vi "3_2_Objects_Detection(Deploy)(Cam).vi"() -> ()   [LabVIEW 2020]
doc: "This example demonstrates usage of Deep Learning Toolkit for object detection based on pretrained network called YOLO https://pjreddie.com/darknet/yolo/\nToolkit's API is utilized to automatically create network architecture based on network topology configuration file and load and initialize network's weights from weight file.\nRequirements: \n1. Deep Learning Toolkit for LabVIEW.\n2. NI Vision Development Module .\n3. Web camera."
uses:
  <vilib>/Ngene/Deep Learning Toolkit/Toolkit/NN_Network/Controls/NN_Device.ctl
  <vilib>/Ngene/Deep Learning Toolkit/Toolkit/NN_Network/Controls/NN_Save_Before_Destroy_Options.ctl
  <vilib>/vision/driver/IMAQdx.llb/IMAQdx Camera Control Mode.ctl
  <vilib>/Ngene/Deep Learning Toolkit/Toolkit/Utils/Vision/Coords_Rect2PolyLine.vi
  <vilib>/Ngene/Deep Learning Toolkit/Toolkit/NN_Network/API/NN_Set_Input/3D/NN_Set_Input(3D_SGL_idx).vi
  <vilib>/Ngene/Deep Learning Toolkit/Toolkit/Deep_Learning_Toolkit_by_Ngene.lvlib
  <vilib>/vision/NI_Vision_Development_Module.lvlib
  <vilib>/vision/driver/NI_Vision_Acquisition_Software.lvlib
  <resource>/objmgr/imaqdx.rc
  <vilib>/ptbypt/NI_PtbyPt.lvlib
panel:
  in  "NN_Device":T1
  out "Speed (FPS)":dbl format="%#_3p"
  out "Loop time(s)":dbl format="%#_3p"
  out "Display":T2(plugin-control)
  in  "Confidence_Thresh":sgl=0.19999999
  in  "IOU_Thresh(NMS)":sgl=0.3
  in  "Stop":bool
  in  "Camera Resolution":i32(listbox)=14
  in  "Camera":refnum<k21>="cam0" caption="IMAQdx Session"
  in  "Model Weights":path=path "D:/Ngene/GitHub/deepltk_examples/3_Image_Processing/33_Object_Detection/Trained Model/512x910_mAP_0.998/Obj_Det_Example_weights_25_06_09__13_45_53.bin"
  in  "Model Topology (CFG)":path=path "D:/Ngene/GitHub/deepltk_examples/3_Image_Processing/33_Object_Detection/Trained Model/512x910_mAP_0.998/Obj_Det_Example_net_cfg_25_06_09__13_45_53.cfg"
  # "Instructions:\n1.Provide the \"Model Topology (CFG)\" and \"Model Weights\" generated after training in \"Objects_Detection(Train).vi\". A pretrained model is also available in the project.\n2. Select the camera from \"Camera\" control.\n3. Run the VI .\n4. Observe the detections drawn on the \"Display\". The info on the top left of each bounding box represents detected object class and the confidence level.\n5. (Optional) Change \"NN_Device\" value to \"GPU\" to compare execution speeds on GPU and CPU.\n\nMore Examples:  https://github.com/ngenehub/deepltk_examples"
  # "Overview:  This example demonstrates the process of deploying an object detection model, capturing samples from a camera, and performing inference.\nRequirements: \n1. Deep Learning Toolkit for LabVIEW.\n2. NI Vision Development Module .\n3. Web camera."
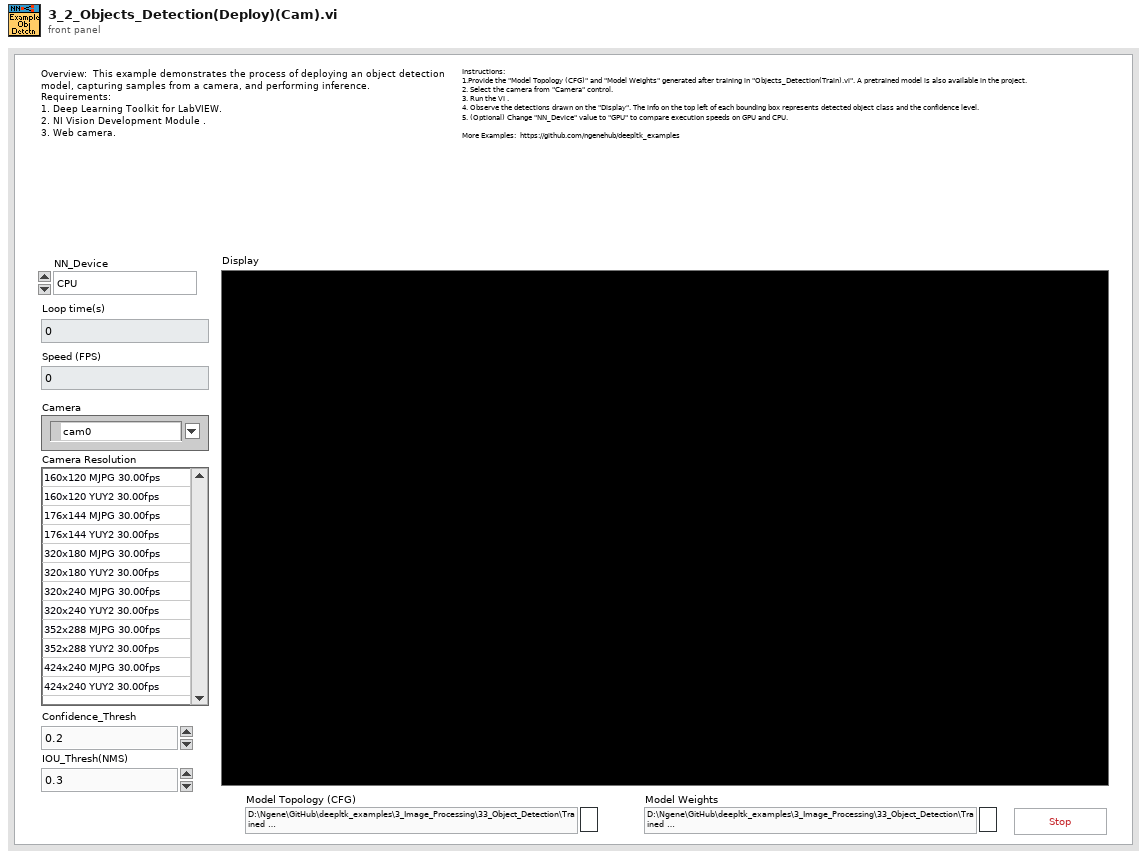
[diagram p1: front panel]
types:
  T1 = typedef "Deep_Learning_Toolkit_by_Ngene.lvlib/NN_Device.ctl" = enum16{"CPU", "GPU"}
  T2 = typedef "IMAQ Image.ctl" = refnum<image>
  T3 = typedef "Deep_Learning_Toolkit_by_Ngene.lvlib/NN_Save_Before_Destroy_Options.ctl" = cluster{"CFG?":bool, "Weights?":bool, "Render?":bool}
  T4 = typedef "NI_Vision_Acquisition_Software.lvlib/IMAQdx Camera Control Mode.ctl" = enum32{"Controller", "Listener"}
  T5 = typedef "Image Type" = u32
  T6 = typedef "IMAQdx.ctl" = refnum<k21>
  T7 = typedef "Deep_Learning_Toolkit_by_Ngene.lvlib/NN_Config_Params.ctl" = cluster{"Name":string, "mBatch":i32, "NN_Train_Params":T8, "LR_Decay_Policy":T11, "Labels":string[], "Loss":T13, "Max_WS_Size(B)":i64, "DryRun?":bool}
  T8 = typedef "Deep_Learning_Toolkit_by_Ngene.lvlib/NN_Train_Params.ctl" = cluster{"Optimizer":T9, "Beta_1":sgl, "Beta_2":sgl, "Weight Decay(L1)":sgl, "Weight Decay(L2)":sgl, "Data_Sampling":T10}
  T9 = typedef "Deep_Learning_Toolkit_by_Ngene.lvlib/NN_Train_Optimizer.ctl" = enum16{"SGD", "Adam", "Adagrad", "Adadelta", "RMSProp", "Nesterov"}
  T10 = typedef "Deep_Learning_Toolkit_by_Ngene.lvlib/NN_Train_Data_Sampling.ctl" = enum16{"Random", "Sequential"}
  T11 = typedef "Deep_Learning_Toolkit_by_Ngene.lvlib/NN_LR_Policy_Cfg.ctl" = cluster{"Policy_Type":T12, "LR0":dbl, "k":sgl, "WarmUp_Policy":enum16{"Step", "Ramp"}, "WarmUp_Iter":i32, "WarmUp_Ratio":sgl}
  T12 = typedef "Deep_Learning_Toolkit_by_Ngene.lvlib/NN_LR_Policy_Type.ctl" = enum16{"Manual", "Step", "Exp", "1/t"}
  T13 = typedef "Deep_Learning_Toolkit_by_Ngene.lvlib/NN_Loss_Config_Params.ctl" = cluster{"Loss_Type":T14, "Loss_Conf_Params":variant}
  T14 = typedef "Deep_Learning_Toolkit_by_Ngene.lvlib/NN_Loss_Type.ctl" = enum16{"None", "MSE", "CrossEntropy", "YOLO_v2", "YOLO_v4"}
  T15 = typedef "Deep_Learning_Toolkit_by_Ngene.lvlib/NN_Layer_Config_Params.ctl" = cluster{"Layer_Type":T16, "Layer_Conf_Params":variant, "Input Layers":string[]}
  T16 = typedef "Deep_Learning_Toolkit_by_Ngene.lvlib/NN_Layer_Type.ctl" = enum16{"Input1D", "Input3D", "Conv1D", "Conv2D", "Conv2D_Adv", "MaxPool", "AvgPool", "UpSample", "DropOut3D", "ShortCut", "Concat", "SoftMax3D", "FC", "DropOut", "Softmax", "Flatten", "YOLO_v2", "YOLO_v4", "Activation", "BatchNormalization", "LayerNormalization", "Scale", "Unsupported"}
  T17 = typedef "Deep_Learning_Toolkit_by_Ngene.lvlib/NN.ctl" = cluster{"Name":string, "No of Layers":i32, "mBatch":i32, "Layers":T18[], "Dimty":T19, "Dims_In":T20, "Dims_Out":T20, "Working_Dir":path, "Train?":bool, "Train_Params":T8, "LR_Update_Policy":T11, "Session Data":T21, "Ground_truth":T22, "NNg_hdls":T23, "NN_Device":T1, "GPU Id":i32, "Labels":string[], "Loss_Type":T14, "Loss_Cfg_Prms":variant, "NNG_WS":T24, "DryRun?":bool}
  T18 = typedef "Deep_Learning_Toolkit_by_Ngene.lvlib/NN_Layer_ref.ctl" = refnum<file>
  T19 = typedef "Deep_Learning_Toolkit_by_Ngene.lvlib/NN_In_Out_Dim-ty.ctl" = enum8{"In1D_Out1D", "In3D_Out1D", "In3D_Out3D", "In3D_OutBBox"}
  T20 = typedef "Deep_Learning_Toolkit_by_Ngene.lvlib/NN_Dims(C,H,W).ctl" = cluster{"C":i32, "H":i32, "W":i32}
  T21 = typedef "Deep_Learning_Toolkit_by_Ngene.lvlib/NN_Train_Session_Data.ctl" = cluster{"Epochs":sgl, "Tot_Iter":i32, "LR":sgl, "LR_iter":i32}
  T22 = typedef "Deep_Learning_Toolkit_by_Ngene.lvlib/NN_Ground_truth.ctl" = cluster{"Y":variant}
  T23 = typedef "Deep_Learning_Toolkit_by_Ngene.lvlib/nng_cuda_handles.ctl" = cluster{"cudnn":u64, "cublas":u64, "stream":u64, "curand":u64}
  T24 = typedef "Deep_Learning_Toolkit_by_Ngene.lvlib/NNG_WS.ctl" = cluster{"NNG_WS_Mem":T25, "Max_WS_Size":i64}
  T25 = typedef "Deep_Learning_Toolkit_by_Ngene.lvlib/NNg_WS_Mem_DVR.ctl" = refnum<data-value>
  T26 = typedef "Deep_Learning_Toolkit_by_Ngene.lvlib/NN_Layer.ctl" = cluster{"Name":string, "Layer_Data":T27, "Layer_Type":T16, "Dims_In":T20, "Layers_In":T18[], "Dims_Out":T20, "Layers_Out":T18[], "Metrics":T28, "GPU_Data":T29, "mBatch":i32, "NN_Device":T1, "NNg_hdls":T23, "Train?":bool, "Dimty":T30, "RecptField":T31, "Idx":i32}
  T27 = typedef "Deep_Learning_Toolkit_by_Ngene.lvlib/NN_Layer_Data_Refnum.ctl" = refnum<file>
  T28 = typedef "Deep_Learning_Toolkit_by_Ngene.lvlib/NN_Layer_Metrics.ctl" = cluster{"Data":dbl, "Params":dbl, "Ops":dbl}
  T29 = typedef "Deep_Learning_Toolkit_by_Ngene.lvlib/NNg_Layer_Data_Refnum.ctl" = refnum<file>
  T30 = typedef "Deep_Learning_Toolkit_by_Ngene.lvlib/NN_Layer_Dimty.ctl" = enum16{"1D", "3D"}
  T31 = typedef "Deep_Learning_Toolkit_by_Ngene.lvlib/NN_Layer_RF_State.ctl" = cluster{"Dims":T32, "J":T32}
  T32 = typedef "Deep_Learning_Toolkit_by_Ngene.lvlib/NN_Dims(V,H).ctl" = cluster{"V":i32, "H":i32}
  T33 = typedef "Deep_Learning_Toolkit_by_Ngene.lvlib/NN_BBox_Detection.ctl" = cluster{"Class":i32, "Conf Level":sgl, "BBox":T34}
  T34 = typedef "Deep_Learning_Toolkit_by_Ngene.lvlib/NN_BBox.ctl" = cluster{"x":sgl, "y":sgl, "w":sgl, "h":sgl}
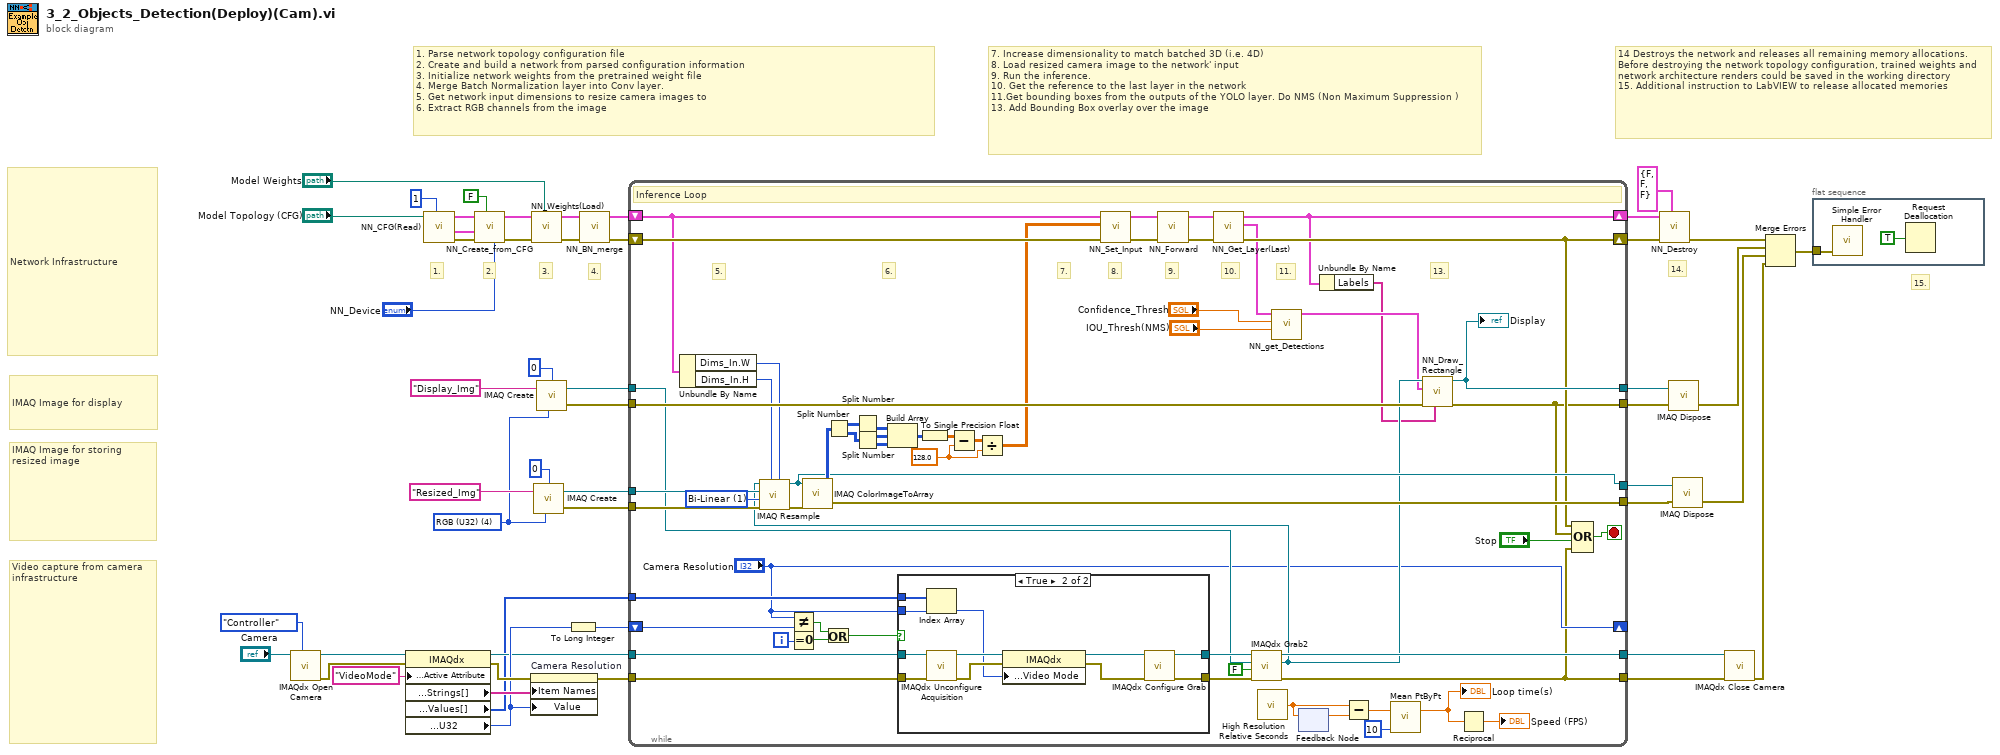
[diagram p0: block diagram]
diagram:
  w16 = T5 4 items=["Grayscale (U8)", "Grayscale (I16)", "Grayscale (SGL)", "Complex (CSG)", "RGB (U32)", "HSL (U32)", "RGB (U64)", "Grayscale (U16)"] ("Image Type")
  # "4."
  # "15."
  # "14 Destroys the network and releases all remaining memory allocations. Before destroying the network topology configuration, trained weights and network architecture renders could be saved in the working directory\n15. Additional instruction to LabVIEW to release allocated memories"
  # "14."
  # "7. Increase dimensionality to match batched 3D (i.e. 4D)\n8. Load resized camera image to the network' input\n9. Run the inference.\n10. Get the reference to the last layer in the network\n11.Get bounding boxes from the outputs of the YOLO layer. Do NMS (Non Maximum Suppression ) \n13. Add Bounding Box overlay over the image"
  # "1. Parse network topology configuration file\n2. Create and build a network from parsed configuration information \n3. Initialize network weights from the pretrained weight file\n4. Merge Batch Normalization layer into Conv layer.\n5. Get network input dimensions to resize camera images to\n6. Extract RGB channels from the image"
  # "Video capture from camera \ninfrastructure"
  # "IMAQ Image for storing \nresized image"
  # "IMAQ Image for display"
  # "Network Infrastructure"
  # "3."
  # "2."
  # "1."
  n1 = call <vilib>:"IMAQdx Open Camera.vi"("Camera Control Mode"=IMAQdx_Camera_Control_Mode."Controller", "Session In"="Camera") -> ("error out"=w27:errorcluster, "Session Out"=w29:T6)  [unwired: 1 in, 7 out]
  n2 = property class="IMAQdx"(reference=w29, error in=w27, "Camera Attributes:Active Attribute"="VideoMode" ("ActiveAttribute")) -> (reference out=w23:T6, error out=w26:errorcluster, "Camera Attributes:Enum:Strings[]"=w25:string[], "Camera Attributes:Enum:Values[]"=w21:u32[], "Camera Attributes:Value:U32"=w24:u32)
  n3 = call <vilib>:"NN_CFG(Read).vi"("mBatch"=1, "CFG file path"="Model Topology (CFG)") -> ("error out"=w47:errorcluster, "Net_Cfg"=w13:T7, "Layer_Cfg"=w48:T15[])  [unwired: 7 in]
  n4 = call <vilib>:"NN_Create_from_CFG.vi"("NN_Device"="NN_Device", "Train? (false)"=FALSE ("Train?"), "error in (no error)"=w47, "Net_Cfg"=w13, "Layer_Cfg"=w48) -> ("error out"=w46:errorcluster, "NN out"=w45:T17)  [unwired: 5 in]
  n5 = property on="Camera Resolution" class="LstBox (strict)"(error in=w26, "Item Names"=w25, "Value"=w24) -> (error out=w20:errorcluster)  [unwired: 1 in, 1 out]
  n6 = call <vilib>:"NN_Weights(Load).vi"("Weight File Path"="Model Weights", "error in (no error)"=w46, "NN in"=w45) -> ("error out"=w5:errorcluster, "NN out"=w3:T17)  [unwired: 7 in]
  n7 = call "IMAQ Create"("Border Size"=0, "Image Name"="Resized_Img", "Image Type"=w16) -> ("New Image"=w34:T2, "error out"=w33:errorcluster)  [unwired: 2 in]
  n8 = call "IMAQ Create"("Border Size"=0, "Image Name"="Display_Img", "Image Type"=w16) -> ("New Image"=w38:T2, "error out"=w41:errorcluster)  [unwired: 2 in]
  n9 = To Long Integer(number=w24) -> (32bit integer=w18:i32)
  n10 = call <vilib>:"NN_BN_merge.vi"("error in (no error)"=w5, "NN in"=w3) -> ("error out"=w4:errorcluster, "NN out"=w2:T17)  [unwired: 8 in]
  n11 = while {
    shift-right: [w53] -> w39
    shift-left: w2 -> [w95]
    shift-right: [w66] -> w40
    shift-left: w4 -> [w102]
    tunnel: [w99] -> w43
    tunnel: [w62] -> w42
    tunnel: w41 -> [w98]
    tunnel: w38 -> [w72]
    tunnel: w34 -> [w96]
    tunnel: w33 -> [w85]
    tunnel: [w83] -> w32
    tunnel: [w82] -> w31
    tunnel: w23 -> [w81]
    tunnel: [w80] -> w22
    tunnel: w21 -> [w74]
    tunnel: w20 -> [w73]
    shift-right: ["Camera Resolution"] -> _
    shift-left: w18 -> [w70]
    tunnel: [w61] -> w11
    i -> [w68]
    stop <- w105 stop-if-true
    w55 = sgl 128.0 ("element")
    w97 = u32 1 items=["Zero Order", "Bi-Linear", "Quadratic", "Cubic Spline"] ("Interpolation Type")
    # "13."
    # "11."
    # "10."
    # "9."
    # "8."
    # "7."
    # "5."
    # "6."
    # "Inference Loop"
    n12 = Unbundle By Name(w95) -> ("Dims_In.W"=w94:i32, "Dims_In.H"=w93:i32)
    n13 = Not Equal?(x="Camera Resolution", y=w70) -> (x != y?=w78:bool)
    n14 = Equal To 0?(x=w68) -> (x = 0?=w77:bool)
    n15 = Or(x=w78, y=w77) -> (x .or. y?=w79:bool)
    n16 = case shown="True" w79 {
      tunnel: w81 -> [w110 w119]
      tunnel: w73 -> [w109 w118]
      tunnel: [w110 w115] -> w75
      tunnel: [w109 w116] -> w76
      tunnel: w74 -> [_ w121]
      tunnel: "Camera Resolution" -> [_ w120]
      frame False {
      }
      frame True {
        n17 = Index Array(array=w121, index=w120) -> (element=w111:u32)
        n18 = call <vilib>:"IMAQdx Unconfigure Acquisition.vi"("error in"=w118, "Session In"=w119) -> ("error out"=w112:errorcluster, "Session Out"=w117:T6)  [unwired: 8 out]
        n19 = property class="IMAQdx"(reference=w117, error in=w112, "Acquisition Attributes:Video Mode"=w111) -> (reference out=w114:T6, error out=w113:errorcluster)
        n20 = call <vilib>:"IMAQdx Configure Grab.vi"("error in"=w113, "Session In"=w114) -> ("error out"=w116:errorcluster, "Session Out"=w115:T6)  [unwired: 2 in, 6 out]
      }
    }
    n21 = call <vilib>:"IMAQdx Grab2.vi"("error in"=w76, "Wait for Next Buffer? (Yes)"=FALSE, "Image In"=w72, "Session In"=w75) -> ("error out"=w61:errorcluster, "Image Out"=w71:T2, "Session Out"=w80:T6)  [unwired: 4 in, 1 out]
    n22 = call "IMAQ Resample"("X Resolution"=w94, "Y Resolution"=w93, "error in (no error)"=w85, "Interpolation Type"=w97, "Image Dst"=w96, "Image Src"=w71) -> ("error out"=w84:errorcluster, "Image Dst Out"=w82:T2)  [unwired: 4 in]
    n23 = call "IMAQ ColorImageToArray"("Image"=w82, "error in (no error)"=w84) -> ("Image Pixels (U32)"=w86:u32[][], "error out"=w83:errorcluster)  [unwired: 2 in, 1 out]
    n24 = Split Number(x=w86) -> (hi(x)=w88:u16[][], lo(x)=w87:u16[][])
    n25 = Split Number(x=w88) -> (lo(x)=w89:u8[][])  [unwired: 1 out]
    n26 = Split Number(x=w87) -> (hi(x)=w90:u8[][], lo(x)=w91:u8[][])
    n27 = Build Array(w89, w90, w91) -> (w92:u8[][][])
    n28 = To Single Precision Float(number=w92) -> (single precision float=w56:sgl[][][])
    n29 = Subtract(x=w56, y=w55) -> (x-y=w57:sgl[][][])
    n30 = Divide(x=w57, y=w55) -> (x/y=w54:sgl[][][])
    n31 = call-poly <vilib>:"NN_Set_Input.vi"("error in (no error)"=w102, "Data_In(3D_SGL)"=w54, "NN in"=w95) -> ("error out"=w100:errorcluster, "NN out"=w101:T17)  [unwired: 7 in]
    n32 = call <vilib>:"NN_Forward.vi"("error in (no error)"=w100, "NN in"=w101) -> ("error out"=w64:errorcluster, "NN out"=w65:T17)  [unwired: 6 in, 2 out]
    n33 = call <vilib>:"NN_Get_Layer(Last).vi"("error in (no error)"=w64, "NN in"=w65) -> ("error out"=w66:errorcluster, "Last_Layer"=w63:T26, "NN out"=w53:T17)  [unwired: 6 in, 1 out]
    n34 = call <vilib>:"High Resolution Relative Seconds.vi"() -> ("relative seconds"=w106:dbl)
    n35 = call <vilib>:"NN_get_Detections.vi"("IOU_Thrsh"="IOU_Thresh(NMS)", "Confidence_Thrsh"="Confidence_Thresh", "YOLO_Layer"=w63) -> ("Detections"=w60:T33[])  [unwired: 7 in, 1 out]
    n36 = feedback #1() -> (w107:dbl)  [unwired: 1 in]
    n37 = feedback-in #1(w106) -> ()
    n38 = Unbundle By Name(w53) -> ("Labels"=w52:string[])
    n39 = Subtract(x=w106, y=w107) -> (x-y=w104:dbl)
    n40 = call <vilib>:"Mean PtByPt.vi"("x"=w104, "sample length"=10) -> ("mean"=w51:dbl)  [unwired: 2 in, 1 out]
    "Loop time(s)" <- w51
    n41 = call "NN_Draw_Rectangle.vi"("Labels"=w52, "error in (no error)"=w98, "Draw_Boxes"=w60, "Img in"=w71) -> ("error out"=w62:errorcluster, "Img out"=w99:T2)  [unwired: 6 in]
    "Display" <- w99
    n42 = Reciprocal(x=w51) -> (1/x=→"Speed (FPS)":dbl)
    n43 = Compound Arithmetic op=OR(w66, w62, "Stop", w61) -> (w105:bool)
  }
  n44 = call <vilib>:"NN_Destroy.vi"("Save (T, T, T)"=T3 {"CFG?"=FALSE, "Weights?"=FALSE, "Render?"=FALSE} ("Save_Config"), "error in (no error)"=w40, "NN in"=w39) -> ("error out"=w49:errorcluster)  [unwired: 7 in, 1 out]
  n45 = call "IMAQ Dispose"("Image"=w43, "error in (no error)"=w42) -> ("error out"=w36:errorcluster)  [unwired: 4 in]
  n46 = call "IMAQ Dispose"("Image"=w31, "error in (no error)"=w32) -> ("error out"=w17:errorcluster)  [unwired: 4 in]
  n47 = call <vilib>:"IMAQdx Close Camera.vi"("error in"=w11, "Session In"=w22) -> ("error out"=w19:errorcluster)  [unwired: 9 out]
  n48 = Merge Errors(w49, w36, w17, w19) -> (w37:errorcluster)
  n49 = flat-sequence {
    tunnel: w37 -> [w122]
    frame #0 {
      n50 = call <vilib>:"Simple Error Handler.vi"("error in (no error)"=w122) -> ()  [unwired: 4 in, 5 out]
      n51 = Request Deallocation(TRUE ("flag")) -> ()
    }
  }
